vi "test-vector-Test1.vi"() -> (3 "All tests passed":bool)   [LabVIEW 2019]
uses:
  <vilib>/Rock Robotics/WPI/ThirdParty/JAS_Junk/TrajLib/VI/CoordAxis_N.vi
  <vilib>/Rock Robotics/WPI/ThirdParty/JAS_Junk/TrajLib/VI/CoordAxis_W.vi
  <vilib>/Rock Robotics/WPI/ThirdParty/JAS_Junk/TrajLib/VI/CoordAxis_U.vi
  <vilib>/Rock Robotics/WPI/ThirdParty/JAS_Junk/TrajLib/VI/CoordSystem_New.vi
  <vilib>/Rock Robotics/WPI/ThirdParty/JAS_Junk/TrajLib/VI/CoordAxis_E.vi
  <vilib>/Rock Robotics/WPI/ThirdParty/JAS_Junk/TrajLib/VI/CoordAxis_D.vi
  <vilib>/Rock Robotics/WPI/ThirdParty/JAS_Junk/TrajLib/Conv_Deg_Radians.vi
  <vilib>/Rock Robotics/WPI/ThirdParty/JAS_Junk/TrajLib/VI/Quaternion_New.vi
  <vilib>/Rock Robotics/WPI/ThirdParty/JAS_Junk/TrajLib/VI/Translation3d_Create.vi
  <vilib>/Rock Robotics/WPI/ThirdParty/JAS_Junk/TrajLib/VI/Pose3d_New_Trans3dRot3d.vi
  <vilib>/Rock Robotics/WPI/ThirdParty/JAS_Junk/TrajLib/VI/Rotation3d_Minus.vi
  <vilib>/Rock Robotics/WPI/ThirdParty/JAS_Junk/TrajLib/VI/Translation3d_Create_Default.vi
  <vilib>/Rock Robotics/WPI/ThirdParty/JAS_Junk/TrajLib/VI/Pose3d_RelativeTo.vi
  <vilib>/Rock Robotics/WPI/ThirdParty/JAS_Junk/TrajLib/VI/Rotation3d_RotateBy.vi
  <vilib>/Rock Robotics/WPI/ThirdParty/JAS_Junk/TrajLib/VI/Translation3d_RotateBy.vi
  <vilib>/Rock Robotics/WPI/ThirdParty/JAS_Junk/TrajLib/VI/Rotation3d_GetQuaterion.vi
  <vilib>/Rock Robotics/WPI/ThirdParty/JAS_Junk/TrajLib/VI/Quaternion_Equals.vi
  <vilib>/Rock Robotics/WPI/ThirdParty/JAS_Junk/TrajLib/VI/CoordAxis_New.vi
  <vilib>/Rock Robotics/WPI/ThirdParty/JAS_Junk/TrajLib/MatBuilder_Create.vi
  <vilib>/Rock Robotics/WPI/ThirdParty/JAS_Junk/TrajLib/Matrix_AssignBlock.vi
  <vilib>/Rock Robotics/WPI/ThirdParty/JAS_Junk/TrajLib/VI/Rotation3D_Create_RotMatrix.vi
  <vilib>/Rock Robotics/WPI/ThirdParty/JAS_Junk/TrajLib/VI/Rotation3d_UnaryMinus.vi
  <vilib>/Rock Robotics/WPI/ThirdParty/JAS_Junk/TrajLib/VI/Transform3d_Create_Pose3dPose3d.vi
  <vilib>/Rock Robotics/WPI/ThirdParty/JAS_Junk/TrajLib/VI/Transform3d_GetRotation3d.vi
  <vilib>/Rock Robotics/WPI/ThirdParty/JAS_Junk/TrajLib/VI/Transform3d_GetTranslation3d.vi
  <vilib>/Rock Robotics/WPI/ThirdParty/JAS_Junk/TrajLib/VI/Rotation3d_Create_Quaternion.vi
  <vilib>/Rock Robotics/WPI/ThirdParty/JAS_Junk/TrajLib/VI/Quaternion_Times.vi
  <vilib>/Rock Robotics/WPI/ThirdParty/JAS_Junk/TrajLib/VI/Quaternion_Inverse.vi
  <vilib>/Rock Robotics/WPI/ThirdParty/JAS_Junk/TrajLib/VI/Quaternion_Get_All.vi
  <vilib>/Rock Robotics/WPI/ThirdParty/JAS_Junk/TrajLib/VI/Quaternion_Get_Vect.vi
  <vilib>/Rock Robotics/WPI/ThirdParty/JAS_Junk/TrajLib/VI/Quaternion_Get_W.vi
  <vilib>/Rock Robotics/WPI/ThirdParty/JAS_Junk/TrajLib/MatrixHelper_CoerceSize.vi
  <vilib>/Rock Robotics/WPI/ThirdParty/JAS_Junk/TrajLib/Matrix_Transpose.vi
  <vilib>/Analysis/baseanly.llb/A x B.vi
  <vilib>/Analysis/baseanly.llb/Real A x B.vi
  <vilib>/Rock Robotics/WPI/ThirdParty/JAS_Junk/TrajLib/Matrix_Ident.vi
  <vilib>/Rock Robotics/WPI/ThirdParty/JAS_Junk/TrajLib/Matrix_IsEqual.vi
  <vilib>/Analysis/baseanly.llb/Determinant.vi
  <vilib>/Analysis/baseanly.llb/Real Determinant.vi
  <vilib>/Rock Robotics/WPI/ThirdParty/JAS_Junk/TrajLib/VI/Transform3d_Create_Trans3dRot3d.vi
  <vilib>/Rock Robotics/WPI/ThirdParty/JAS_Junk/TrajLib/VI/Translation3d_Minus.vi
  <vilib>/Rock Robotics/WPI/ThirdParty/JAS_Junk/TrajLib/VI/Quaternion_Normalize.vi
  <vilib>/Rock Robotics/WPI/ThirdParty/JAS_Junk/TrajLib/VI/Quaternion_New_Default.vi
  <vilib>/Analysis/Matrix/Numeric/Conversions/Array To Matrix.vi
  <vilib>/Analysis/Matrix/Numeric/Conversions/Array To Matrix - RA.vi
  <vilib>/Analysis/7linalg.llb/Create Special Matrix.vi
  <vilib>/Analysis/7linalg.llb/Create Special Real Matrix.vi
  <vilib>/Rock Robotics/WPI/ThirdParty/JAS_Junk/TrajLib/Trajectory_Library.lvlib
panel:
  out "Test 4":bool
  out "Test 3":bool
  out "Test 2":bool
  out "Test 1":bool
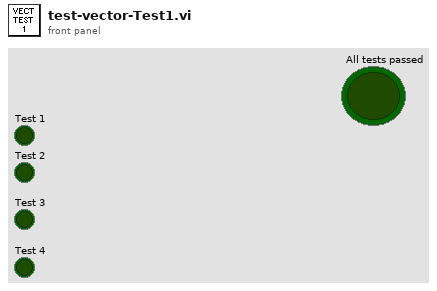
[diagram p1: front panel]
types:
  T1 = typedef "NI_Matrix.lvlib/RealMatrix.ctl" = dbl[][]
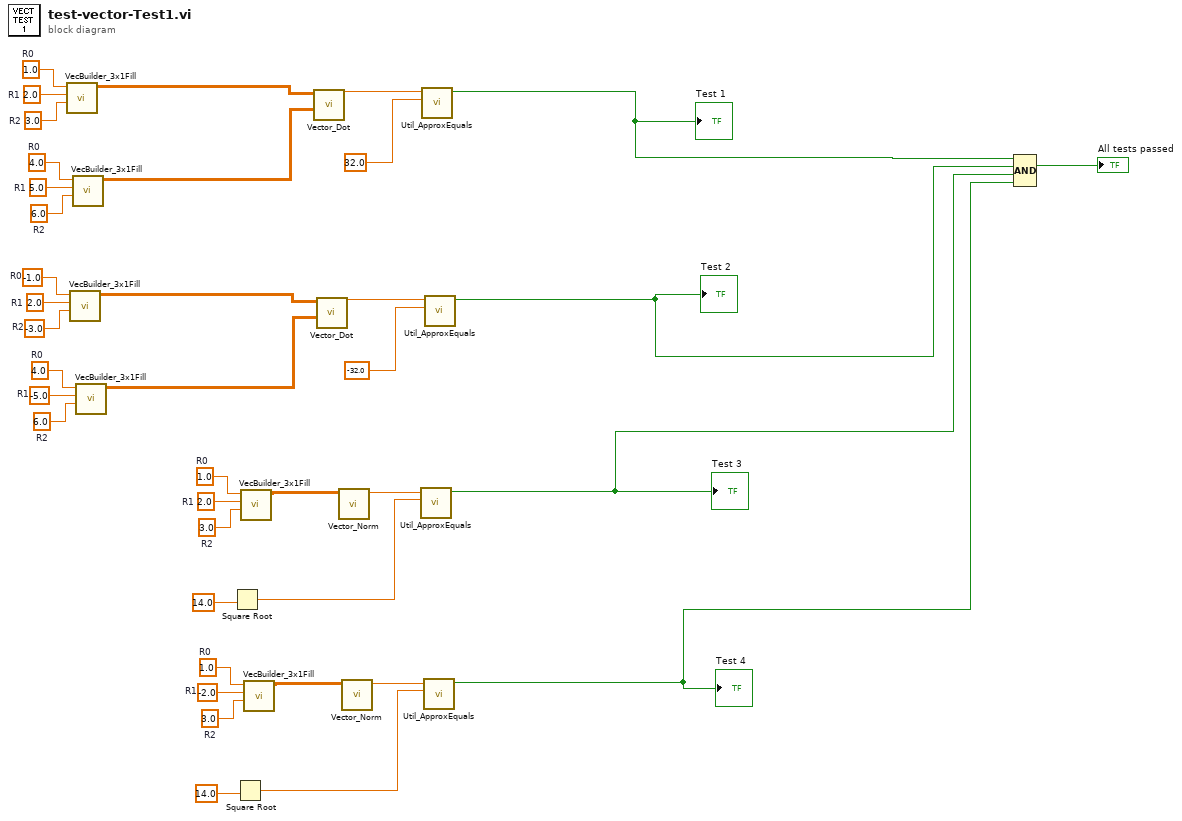
[diagram p0: block diagram]
diagram:
  w11 = 3.0  # R2
  w10 = -2.0  # R1
  w9 = 1.0  # R0
  w18 = 3.0  # R2
  w17 = 2.0  # R1
  w16 = 1.0  # R0
  w25 = 6.0  # R2
  w24 = -5.0  # R1
  w23 = 4.0  # R0
  w28 = -3.0  # R2
  w27 = 2.0  # R1
  w26 = -1.0  # R0
  w35 = 6.0  # R2
  w34 = 5.0  # R1
  w33 = 4.0  # R0
  w38 = 3.0  # R2
  w37 = 2.0  # R1
  w36 = 1.0  # R0
  n1 = call <vilib>:"VecBuilder_3x1Fill.vi"("R2"=w38, "R1"=w37, "R0"=w36) -> ("output matrix"=w32:T1)  [unwired: 8 in]
  n2 = call <vilib>:"VecBuilder_3x1Fill.vi"("R2"=w28, "R1"=w27, "R0"=w26) -> ("output matrix"=w22:T1)  [unwired: 8 in]
  n3 = call <vilib>:"VecBuilder_3x1Fill.vi"("R2"=w35, "R1"=w34, "R0"=w33) -> ("output matrix"=w31:T1)  [unwired: 8 in]
  n4 = call <vilib>:"VecBuilder_3x1Fill.vi"("R2"=w25, "R1"=w24, "R0"=w23) -> ("output matrix"=w21:T1)  [unwired: 8 in]
  n5 = Square Root(x=14.0) -> (sqrt(x)=w12:dbl)
  n6 = Square Root(x=14.0) -> (sqrt(x)=w5:dbl)
  n7 = call <vilib>:"VecBuilder_3x1Fill.vi"("R2"=w18, "R1"=w17, "R0"=w16) -> ("output matrix"=w15:T1)  [unwired: 8 in]
  n8 = call <vilib>:"VecBuilder_3x1Fill.vi"("R2"=w11, "R1"=w10, "R0"=w9) -> ("output matrix"=w8:T1)  [unwired: 8 in]
  n9 = call <vilib>:"Vector_Dot.vi"("Input Vector 2"=w31, "Input Vector 1"=w32) -> ("dot product"=w30:dbl)  [unwired: 9 in]
  n10 = call <vilib>:"Vector_Dot.vi"("Input Vector 2"=w21, "Input Vector 1"=w22) -> ("dot product"=w20:dbl)  [unwired: 9 in]
  n11 = call <vilib>:"Vector_Norm.vi"("Input Vector"=w15) -> ("norm"=w13:dbl)  [unwired: 10 in]
  n12 = call <vilib>:"Vector_Norm.vi"("Input Vector"=w8) -> ("norm"=w6:dbl)  [unwired: 10 in]
  n13 = call <vilib>:"Util_ApproxEquals.vi"("Value 2"=w12, "Value 1"=w13) -> ("ApproxEquals"=w2:bool)  [unwired: 9 in]
  "Test 3" <- w2
  n14 = call <vilib>:"Util_ApproxEquals.vi"("Value 2"=32.0, "Value 1"=w30) -> ("ApproxEquals"=w4:bool)  [unwired: 9 in]
  "Test 1" <- w4
  n15 = call <vilib>:"Util_ApproxEquals.vi"("Value 2"=w5, "Value 1"=w6) -> ("ApproxEquals"=w1:bool)  [unwired: 9 in]
  "Test 4" <- w1
  n16 = call <vilib>:"Util_ApproxEquals.vi"("Value 2"=-32.0, "Value 1"=w20) -> ("ApproxEquals"=w3:bool)  [unwired: 9 in]
  "Test 2" <- w3
  n17 = Compound Arithmetic op=AND(w4, w3, w2, w1) -> (→"All tests passed":bool)
